vi "Read From PWM Camera.vi"() -> (0 "Distance":dbl, 1 "Angle":dbl, 2 "Is Detected?":bool)   [LabVIEW 2016]
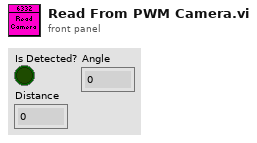
[diagram p1: front panel]
types:
  T1 = typedef "WPI_DigitalInputDevRef.ctl" = cluster{"DevStatus":errorcluster, "DIO Channel":T2}
  T2 = typedef "FPGA_DIOChannel.ctl" = enum8{"DIO 0", "DIO 1", "DIO 2", "DIO 3", "DIO 4", "DIO 5", "DIO 6", "DIO 7", "DIO 8", "DIO 9", "DIO MXP 0", "DIO MXP 1", "DIO MXP 2", "DIO MXP 3", "DIO MXP 4", "DIO MXP 5", "DIO MXP 6", "DIO MXP 7", "DIO MXP 8", "DIO MXP 9", "DIO MXP 10", "DIO MXP 11", "DIO MXP 12", "DIO MXP 13", "DIO MXP 14", "DIO MXP 15", "SPI Port CS1", "SPI Port CS2", "SPI Port CS3", "SPI Port MISO", "SPI Port MOSI", "Invalid"}
  T3 = typedef "WPI_AnalogChannelDevRef.ctl" = cluster{"DevStatus":errorcluster, "Analog Channel":T4}
  T4 = typedef "FPGA_AIChannel.ctl" = enum8{"AI 0", "AI 1", "AI 2", "AI 3", "AI MXP 0", "AI MXP 1", "AI MXP 2", "AI MXP 3", "Invalid"}
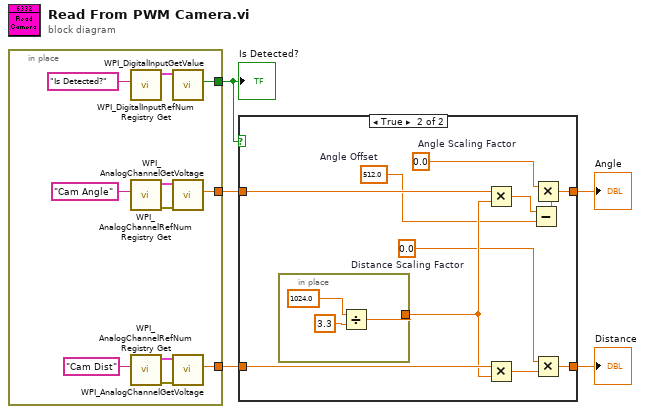
[diagram p0: block diagram]
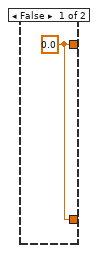
[diagram p2: hidden frame]
diagram:
  n1 = in-place {
    in-place-border: [w8] -> w3
    in-place-border: [w7] -> w5
    in-place-border: [w6] -> w4
    n2 = call <vilib>:"WPI_DigitalInputRefNum Registry Get.vi"("refnum name"="Is Detected?") -> ("DigitalInputDevRef"=w9:T1)  [unwired: 9 in, 1 out]
    n3 = call <vilib>:"WPI_AnalogChannelRefNum Registry Get.vi"("refnum name"="Cam Angle") -> ("error out"=w16:errorcluster, "AIDeviceRef"=w15:T3)  [unwired: 9 in]
    n4 = call <vilib>:"WPI_AnalogChannelRefNum Registry Get.vi"("refnum name"="Cam Dist") -> ("error out"=w13:errorcluster, "AIDeviceRef"=w14:T3)  [unwired: 9 in]
    n5 = call <vilib>:"WPI_DigitalInputGetValue.vi"("DigitalInputDevRef"=w9) -> ("Value"=w8:bool)  [unwired: 8 in, 2 out]
    n6 = call <vilib>:"WPI_AnalogChannelGetVoltage.vi"("error in (no error)"=w16, "AIDeviceRef"=w15) -> ("Voltage"=w6:dbl)  [unwired: 7 in, 2 out]
    n7 = call <vilib>:"WPI_AnalogChannelGetVoltage.vi"("error in (no error)"=w13, "AIDeviceRef"=w14) -> ("Voltage"=w7:dbl)  [unwired: 7 in, 2 out]
  }
  "Is Detected?" <- w3
  n8 = case shown="True" w3 {
    tunnel: w5 -> [_ w28]
    tunnel: w4 -> [_ w27]
    tunnel: [w17 w22] -> w2
    tunnel: [w17 w21] -> w1
    frame False {
      w17 = 0.0
    }
    frame True {
      w18 = 512.0  # Angle Offset
      w23 = 0.0  # Angle Scaling Factor
      w24 = 0.0  # Distance Scaling Factor
      n9 = in-place {
        in-place-border: [w29] -> w26
        n10 = Divide(x=1024.0 ("x*y"), y=3.3) -> (x/y=w29:dbl)
      }
      n11 = Multiply(x=w27, y=w26) -> (x*y=w19:dbl)
      n12 = Multiply(x=w28, y=w26) -> (x*y=w25:dbl)
      n13 = Subtract(x=w19, y=w18) -> (x-y=w20:dbl)
      n14 = Multiply(x=w23, y=w20) -> (x*y=w21:dbl)
      n15 = Multiply(x=w24, y=w25) -> (x*y=w22:dbl)
    }
  }
  "Distance" <- w2
  "Angle" <- w1
